vi "AmplitudeModulation.vi"() -> ()   [LabVIEW 2016]
uses:
  <vilib>/DAQmx/read.llb/DAQmx Read (Analog 1D DBL NChan 1Samp).vi
  <vilib>/DAQmx/miscellaneous.llb/DAQmx Fill In Error Info.vi
  <vilib>/addons/control/pid/pid.llb/PID (DBL).vi
  <instrlib>/Agilent 33XXX Series/Agilent 33XXX Series.lvlib
  <vilib>/addons/control/pid/NI_PID_pid.lvlib
  <vilib>/ptbypt/NI_PtbyPt.lvlib
panel:
  in  "View Saved Data\nUpon Completion":bool=TRUE
  out "Time Elapsed (s)":u32
  out "Temperature":dbl[](graph) caption="Signals"
  in  "Slide":dbl(slide) scale=35.0..45.0
  in  "Start":bool
  out "Actual Samp\nRate (Hz)":dbl format="%#_2g"
  in  "Feed back Mechanism":enum32{"PID Control", "Simple P Control"}(tab)
  in  "PID gains":T1={"proportional gain (Kc)"=0.03, "integral time (Ti, min)"=0.175, "derivative time (Td, min)"=0.002} {"derivative time (Td, min)" format="%.3f"; "integral time (Ti, min)" format="%.3f"; "proportional gain (Kc)" format="%.3f"}
  in  "Simple P":dbl
  in  "Amplitude\nModulation?":bool=TRUE
  in  "voltage limit":dbl=0.95 format="%#_13g"
  in  "Set Point (C)":dbl=40.0
  in  "Total Time (s)":u32=300
  in  "Output":bool=TRUE
  in  "Amplitude (V)":dbl=0.2 format="%#_3g"
  in  "Stop":bool
  out "Current Reading":dbl=34.489131869267396 format="%#.1g"
  out "Waveform Chart":waveform(dbl)(graph)
  in  "Log Data?":bool=TRUE
  in  "Description":string="Test Data. See Pictures."
  in  "File Path":path=path "C:/Data/Sonify Labview/ChickenWithChillerWithStandoff.lvm" caption="Filename"
  # "(Set Point - Current Reading) * P\n+ Current Voltage\n= New Voltage"
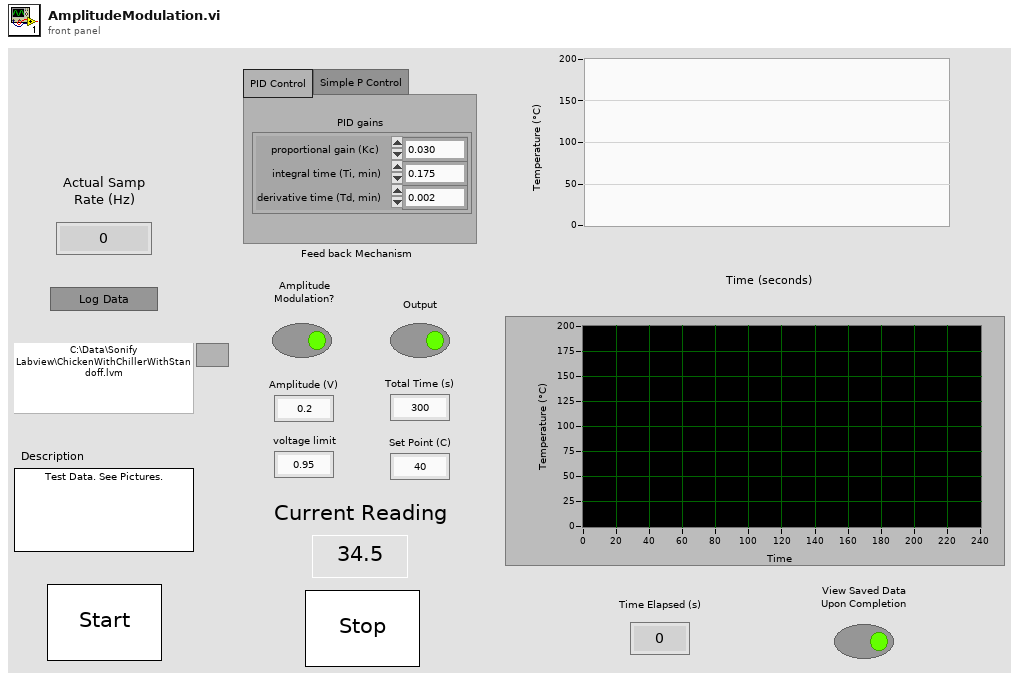
[diagram p1: front panel]
types:
  T1 = cluster{"proportional gain (Kc)":dbl, "integral time (Ti, min)":dbl, "derivative time (Td, min)":dbl}
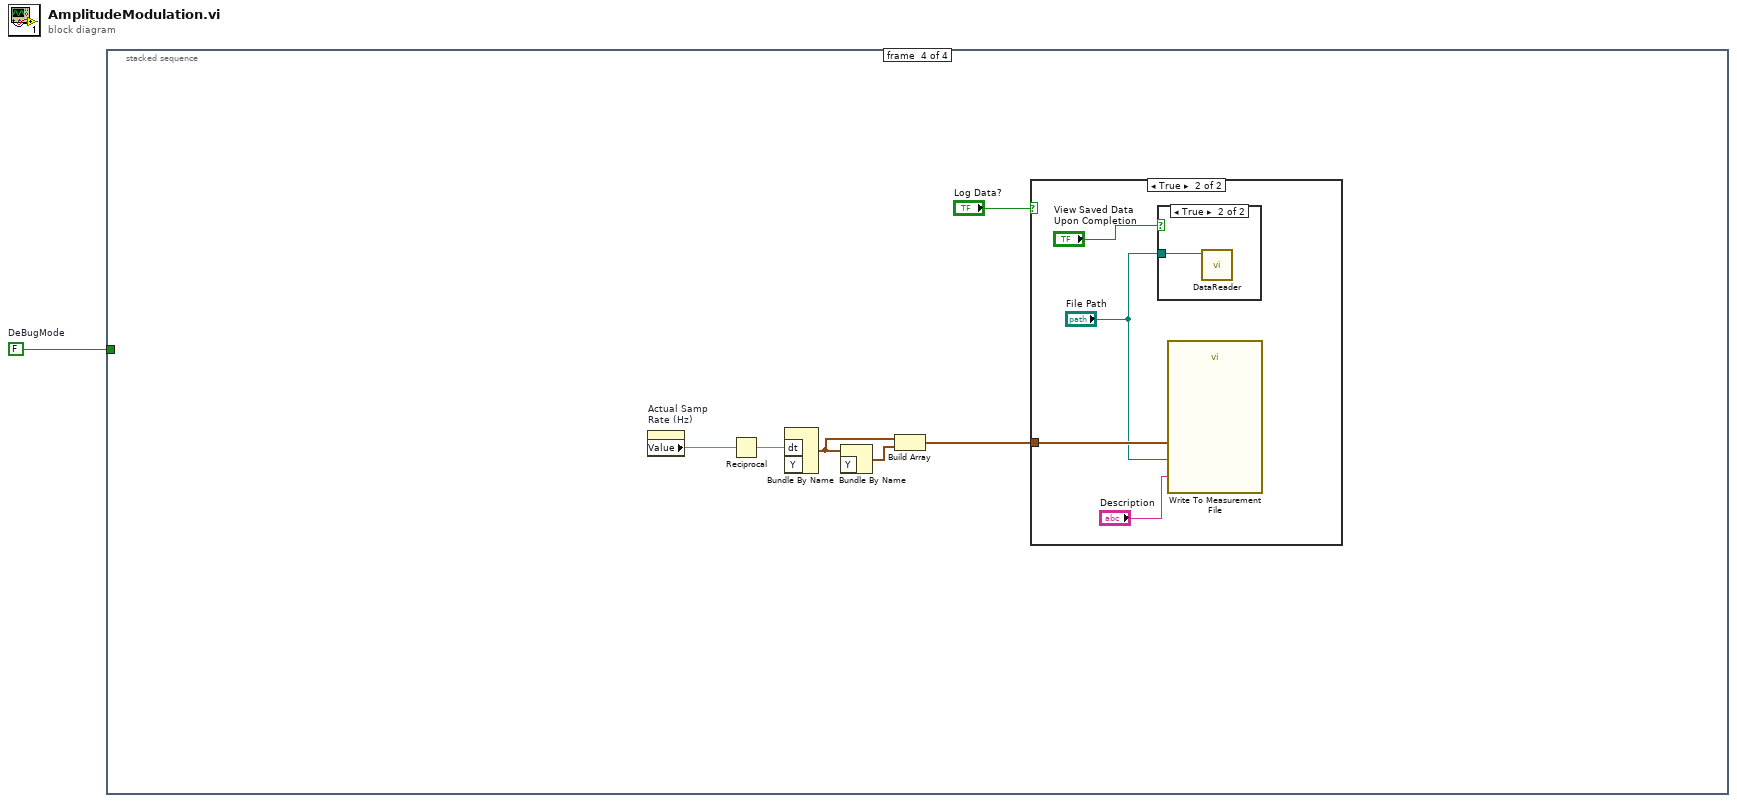
[diagram p0: block diagram]
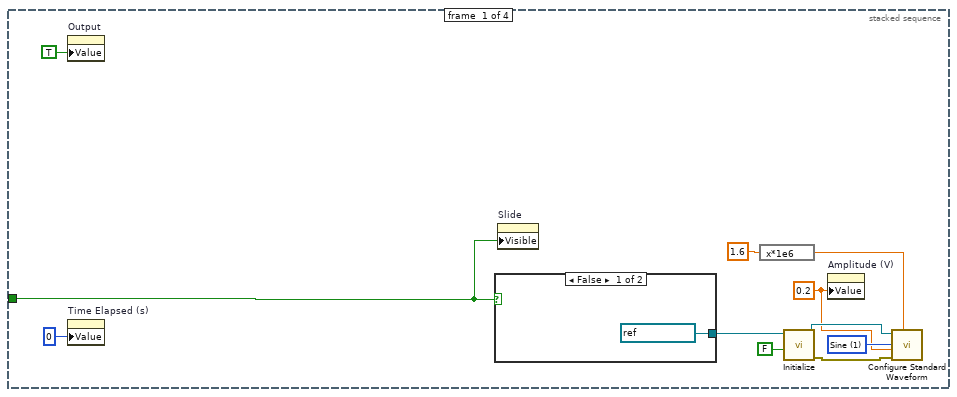
[diagram p2: hidden frame]
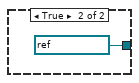
[diagram p3: hidden frame]
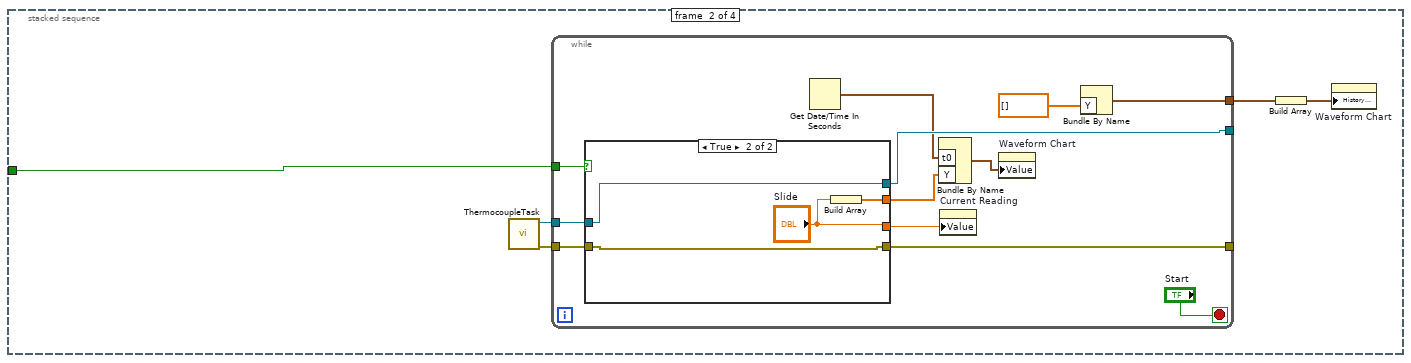
[diagram p4: hidden frame]
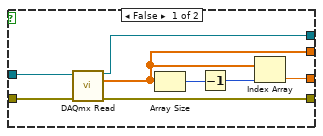
[diagram p5: hidden frame]
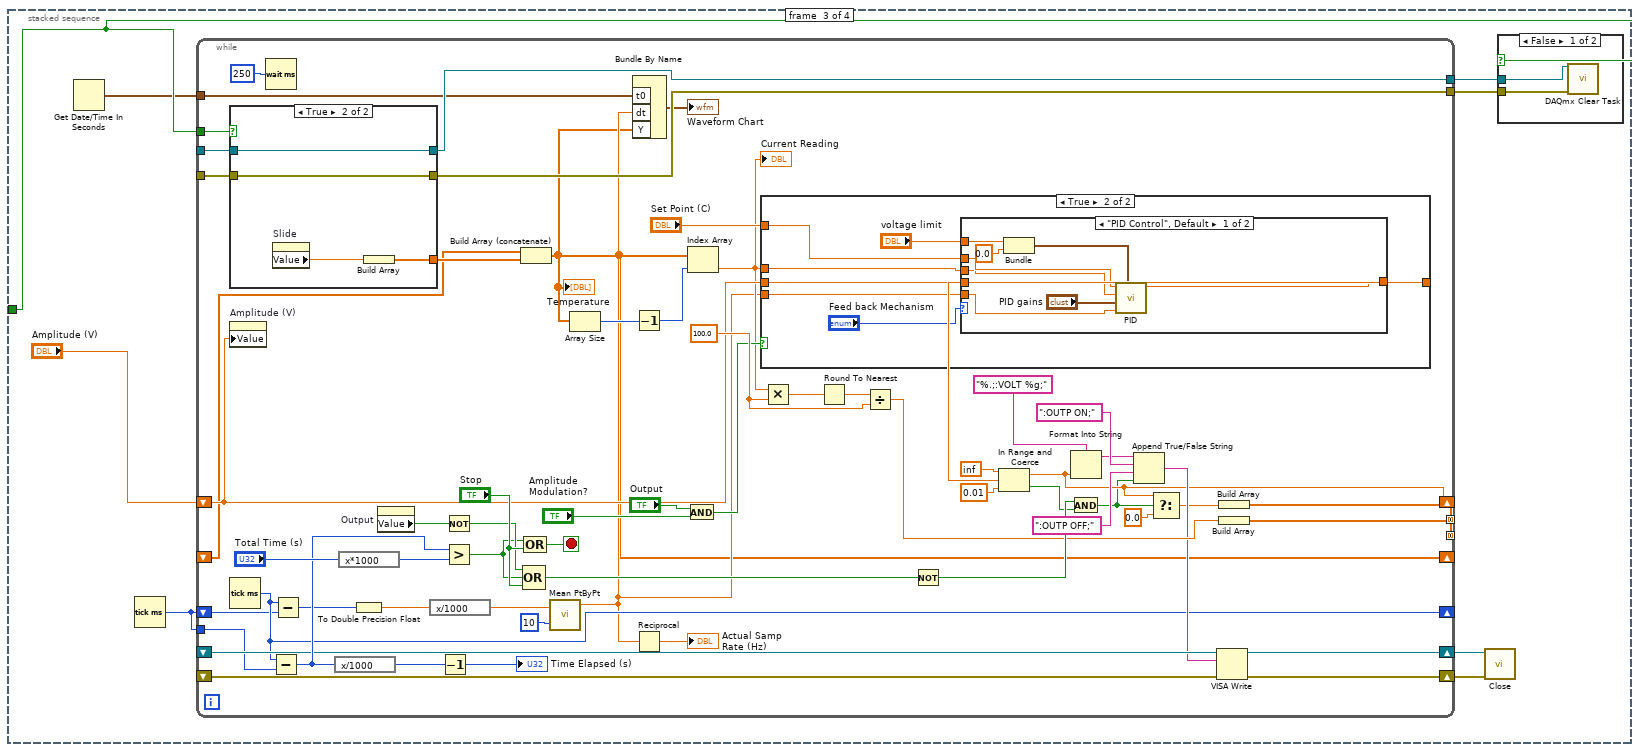
[diagram p6: hidden frame]
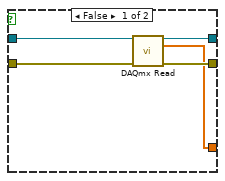
[diagram p8: hidden frame]
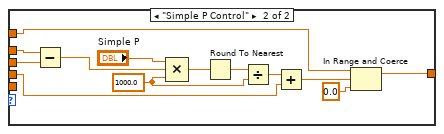
[diagram p10: hidden frame]
diagram:
  w1 = FALSE  # DeBugMode
  n1 = stacked-sequence {
    seq-local: [_ _ w59 _] -> [_ _ _ w171]
    seq-local: [w6 _ _ _] -> [_ _ w55 _]
    seq-local: [w5 _ _ _] -> [_ _ w54 _]
    seq-local: [_ w21 _ _] -> [_ _ w52 _]
    seq-local: [_ w20 _ _] -> [_ _ w51 _]
    seq-local: [_ _ w50 _] -> [_ _ _ w169]
    tunnel: w1 -> [w2 w17 w49 _]
    frame #0 {
      w8 = u16 1 items=["DC", "Sine", "Square", "Triangle", "Ramp", "Pulse", "Noise", "Sinc", "Negative Ramp", "Exponential Rise", "Exponential Fall", "Cardiac"] ("Waveform Function (1: Sine)")
      w3 = 0.2 ("Amplitude (1)")
      n2 = property on="Output" class="Bool (strict)"("Value"=TRUE ("Enable Output  (T: Enable)")) -> ()  [unwired: 2 in, 2 out]
      n3 = property on="Time Elapsed (s)" class="DigNum (strict)"("Value"=u32 0 ("Time Elapsed (s)")) -> ()  [unwired: 2 in, 2 out]
      n4 = case shown="False" w2 {
        tunnel: [refnum<visa-resource-name> "FunGen1" ("Function Gen Address") refnum<visa-resource-name> "FunGen2" ("Function Gen Address")] -> w12
        frame False {
        }
        frame True {
        }
      }
      n5 = property on="Slide" class="Slide (strict)"("Visible"=w2) -> ()  [unwired: 2 in, 2 out]
      n6 = expression code="x*1e6"(1.6 ("Frequency (1000 Hz)")) -> (w4:dbl)
      n7 = call <instrlib>:"Initialize.vi"("Reset (True)"=FALSE, "VISA resource name"=w12) -> ("error out"=w10:errorcluster, "VISA resource name out"=w11:refnum<visa-resource-name>)  [unwired: 8 in]
      n8 = property on="Amplitude (V)" class="DigNum (strict)"("Value"=w3) -> ()  [unwired: 2 in, 2 out]
      n9 = call <instrlib>:"Configure Standard Waveform.vi"("Frequency (1000 Hz)"=w4, "error in (no error)"=w10, "Amplitude (1)"=w3, "Waveform Function (1: Sine)"=w8, "VISA resource name"=w11) -> ("error out"=w5:errorcluster, "VISA resource name out"=w6:refnum<visa-resource-name>)  [unwired: 5 in]
    }
    frame #1 {
      n10 = call "ThermocoupleTask.vi"() -> ("error out"=w22:errorcluster, "task out"=w23:refnum<k21>)  [unwired: 10 in]
      n11 = while {
        tunnel: w23 -> [w35]
        tunnel: w22 -> [w34]
        tunnel: [w30] -> w21
        tunnel: [w29] -> w20
        tunnel: [w27] -> w19
        tunnel: w17 -> [w25]
        stop <- "Start" stop-if-true
        n12 = case shown="True" w25 {
          tunnel: w35 -> [w43 w47]
          tunnel: w34 -> [w42 w46]
          tunnel: [w39 w44] -> w32
          tunnel: [w38 "Slide"] -> w31
          tunnel: [w37 w47] -> w30
          tunnel: [w36 w46] -> w29
          frame False {
            n13 = call-poly <vilib>:"DAQmx Read.vi"("task/channels in"=w43, "error in"=w42) -> ("task out"=w37:refnum<k21>, "data"=w39:dbl[], "error out"=w36:errorcluster)  [unwired: 11 in]
            n14 = Array Size(array=w39) -> (size(s)=w41:i32)
            n15 = Decrement(x=w41) -> (x-1=w40:i32)
            n16 = Index Array(array=w39, index=w40) -> (element=w38:dbl)
          }
          frame True {
            n17 = Build Array("Slide") -> (w44:dbl[])
          }
        }
        n18 = Get Date/Time In Seconds() -> (seconds since 1Jan1904=w24:timestamp)
        n19 = Bundle By Name("t0"=w24, "Y"=w32) -> (w28:waveform(dbl))  [unwired: 1 in]
        n20 = property on="Current Reading" class="DigNum (strict)"("Value"=w31) -> ()  [unwired: 2 in, 2 out]
        n21 = property on="Waveform Chart" class="WFChart (strict)"("Value"=w28) -> ()  [unwired: 2 in, 2 out]
        n22 = Bundle By Name("Y"=dbl[] []) -> (w27:waveform(dbl))  [unwired: 1 in]
      }
      n23 = Build Array(w19) -> (w18:waveform(dbl)[])
      n24 = property on="Waveform Chart" class="WFChart (strict)"("History Data"=w18) -> ()  [unwired: 2 in, 2 out]
    }
    frame #2 {
      n25 = Get Date/Time In Seconds() -> (seconds since 1Jan1904=w48:timestamp)
      n26 = Tick Count (ms)() -> (millisecond timer value=w56:u32)
      n27 = while {
        shift-right: [w103] -> w61
        shift-left: w54 -> [w101]
        shift-right: [w104] -> w60
        shift-left: w55 -> [w102]
        tunnel: w56 -> [w94]
        shift-right: [w75] -> _
        shift-left: "Amplitude (V)" -> [w100]
        tunnel: [w118] -> w59 mode=concatenating
        shift-right: [w85] -> _
        shift-left: w56 -> [w84]
        tunnel: w52 -> [w90]
        tunnel: [w89] -> w58
        tunnel: [w88] -> w57
        tunnel: w51 -> [w87]
        tunnel: [w71] -> w50 mode=concatenating
        tunnel: w49 -> [w68]
        shift-right: [w65] -> _
        shift-left: _ -> [w66]
        tunnel: w48 -> [w64]
        stop <- w126 stop-if-true
        w114 = 100.0 ("y")
        n28 = case shown="True" w68 {
          tunnel: w90 -> [w131 w133]
          tunnel: [w130 w133] -> w89
          tunnel: [w129 w132] -> w88
          tunnel: w87 -> [w128 w132]
          tunnel: [w127 w134] -> w67
          frame False {
            n29 = call-poly <vilib>:"DAQmx Read.vi"("task/channels in"=w131, "error in"=w128) -> ("task out"=w130:refnum<k21>, "data"=w127:dbl[], "error out"=w129:errorcluster)  [unwired: 11 in]
          }
          frame True {
            n30 = property on="Slide" class="Slide (strict)"() -> ("Value"=w135:dbl)  [unwired: 2 in, 2 out]
            n31 = Build Array(w135) -> (w134:dbl[])
          }
        }
        n32 = property on="Amplitude (V)" class="DigNum (strict)"("Value"=w100) -> ()  [unwired: 2 in, 2 out]
        n33 = Tick Count (ms)() -> (millisecond timer value=w85:u32)
        n34 = Wait (ms)(milliseconds to wait=u32 250) -> ()  [unwired: 1 out]
        n35 = Subtract(x=w85, y=w94) -> (x-y=w106:u32)
        n36 = Subtract(x=w85, y=w84) -> (x-y=w83:u32)
        n37 = expression code="x/1000"(w106) -> (w78:u32)
        n38 = expression code="x*1000"("Total Time (s)") -> (w124:u32)
        n39 = To Double Precision Float(number=w83) -> (double precision float=w80:dbl)
        n40 = property on="Output" class="Bool (strict)"() -> ("Value"=w120:bool)  [unwired: 2 in, 2 out]
        n41 = expression code="x/1000"(w80) -> (w82:dbl)
        n42 = Decrement(x=w78) -> (x-1=→"Time Elapsed (s)":u32)
        n43 = Not(x=w120) -> (.not. x?=w113:bool)
        n44 = Greater?(x=w106, y=w124) -> (0:w112:bool)
        n45 = Build Array (concatenate)(w66, w67) -> (w65:dbl[])
        "Temperature" <- w65
        n46 = Compound Arithmetic op=OR(w113, w112, "Stop") -> (w122:bool)
        n47 = Compound Arithmetic op=OR(w112, "Stop") -> (w126:bool)
        n48 = call <vilib>:"Mean PtByPt.vi"("x"=w82, "sample length"=10) -> ("mean"=w69:dbl)  [unwired: 2 in, 1 out]
        n49 = Array Size(array=w65) -> (size(s)=w92:i32)
        n50 = Bundle By Name("t0"=w64, "dt"=w69, "Y"=w65) -> (→"Waveform Chart":waveform(dbl))  [unwired: 1 in]
        n51 = Decrement(x=w92) -> (x-1=w91:i32)
        n52 = Reciprocal(x=w69) -> (1/x=→"Actual Samp\nRate (Hz)":dbl)
        n53 = And(x="Output", y="Amplitude\nModulation?") -> (x .and. y?=w107:bool)
        n54 = Index Array(array=w65, index=w91) -> (element=w93:dbl)
        "Current Reading" <- w93
        n55 = case shown="True" w107 {
          tunnel: w93 -> [_ w142]
          tunnel: [w136 w140] -> w105
          tunnel: w100 -> [w136 w141]
          tunnel: "Set Point (C)" -> [_ w143]
          tunnel: w69 -> [_ w138]
          frame False {
          }
          frame True {
            n56 = case shown="\"PID Control\", Default" "Feed back Mechanism" {
              tunnel: w143 -> [w147 w161]
              tunnel: w142 -> [w145 w160]
              tunnel: w141 -> [_ w158]
              tunnel: [w148 w155] -> w140
              tunnel: "voltage limit" -> [w146 w157]
              tunnel: w138 -> [w144 _]
              frame "PID Control", Default {
                n57 = Bundle("voltage limit"=w146, "output low"=0.0) -> (w151:cluster{"voltage limit":dbl, "output low":dbl})  [unwired: 1 in]
                n58 = call-poly <vilib>:"PID.vi"("output range"=w151, "dt (s)"=w144, "PID gains"="PID gains", "process variable"=w145, "setpoint"=w147) -> ("output"=w148:dbl)  [unwired: 5 in, 1 out]
              }
              frame "Simple P Control" {
                w162 = 1000.0 ("y")
                n59 = Subtract(x=w161, y=w160) -> (x-y=w153:dbl)
                n60 = Compound Arithmetic op=MULTIPLY("Simple P", w153, w162) -> (w164:dbl)
                n61 = Round To Nearest(number=w164) -> (nearest integer value=w163:dbl)
                n62 = Divide(x=w163, y=w162) -> (x/y=w159:dbl)
                n63 = Add(x=w159, y=w158) -> (x+y=w156:dbl)
                n64 = In Range and Coerce(upper limit=w157, x=w156, lower limit=0.0) -> (coerced(x)=w155:dbl)  [unwired: 1 out]
              }
            }
          }
        }
        n65 = Multiply(x=w93, y=w114) -> (x*y=w117:dbl)
        n66 = Round To Nearest(number=w117) -> (nearest integer value=w116:dbl)
        n67 = Divide(x=w116, y=w114) -> (x/y=w115:dbl)
        n68 = Not(x=w122) -> (.not. x?=w123:bool)
        n69 = In Range and Coerce(upper limit=inf, x=w105, lower limit=0.01) -> (coerced(x)=w75:dbl, In Range?=w108:bool)
        n70 = Format Into String(format string="%.;:VOLT %g;" ("Amplitude Command"), w75) -> (resulting string=w96:string)  [unwired: 2 in, 1 out]
        n71 = And(x=w123, y=w108) -> (x .and. y?=w73:bool)
        n72 = Append True/False String(1:w73, 2:":OUTP OFF;" ("true string"), 3:":OUTP ON;" ("true string"), 4:w96) -> (0:w95:string)
        n73 = Select(t=w75, s=w73, f=0.0) -> (s? t:f=w72:dbl)
        n74 = VISA Write(VISA resource name=w102, write buffer=w95, error in (no error)=w101) -> (VISA resource name out=w104:refnum<visa-resource-name>, error out=w103:errorcluster)  [unwired: 1 out]
        n75 = Build Array(w72) -> (w71:dbl[])
        n76 = Build Array(w115) -> (w118:dbl[])
      }
      n77 = call <instrlib>:"Close.vi"("error in (no error)"=w61, "VISA resource name"=w60) -> ()  [unwired: 9 in, 1 out]
      n78 = case shown="False" w49 {
        tunnel: w58 -> [w63 _]
        tunnel: w57 -> [w62 _]
        frame False {
          n79 = call <vilib>:"DAQmx Clear Task.vi"("task in"=w63, "error in"=w62) -> ()  [unwired: 13 in, 1 out]
        }
        frame True {
        }
      }
    }
    frame #3 {
      n80 = property on="Actual Samp\nRate (Hz)" class="DigNum (strict)"() -> ("Value"=w170:dbl)  [unwired: 2 in, 2 out]
      n81 = Reciprocal(x=w170) -> (1/x=w165:dbl)
      n82 = Bundle By Name("dt"=w165, "Y"=w171) -> (w166:waveform(dbl))  [unwired: 1 in]
      n83 = Bundle By Name(cluster=w166, "Y"=w169) -> (w168:waveform(dbl))
      n84 = Build Array(w166, w168) -> (w167:waveform(dbl)[])
      n85 = case shown="True" "Log Data?" {
        tunnel: w167 -> [_ w175]
        frame False {
        }
        frame True {
          n86 = case shown="True" "View Saved Data\nUpon Completion" {
            tunnel: "File Path" -> [_ w177]
            frame False {
            }
            frame True {
              n87 = call "DataReader.vi"("Filename"=w177) -> ()  [unwired: 11 in]
            }
          }
          n88 = call "Write To Measurement File"("Signals"=w175, "Filename"="File Path", "Comment"="Description") -> ()  [unwired: 14 in, 3 out]
        }
      }
    }
  }
